vi "Read Cooler ON_OFF.vi"(8 "error in (no error)":errorcluster, 11 "CCDCamera in":refnum<class "Simulated_CCD_Camera.lvclass">) -> (0 "error out":errorcluster, 2 "COOLER_POWER_STATUS":u16, 3 "CCDCamera out":refnum<class "Simulated_CCD_Camera.lvclass">)   [LabVIEW 2018, in "Simulated_CCD_Camera.lvclass"]
uses:
  Simulated_CCD_Camera.lvclass
  Simulated_CCD_Camera.lvclass/Simulated_CCD_Camera.ctl
  Interface/Interface.lvclass
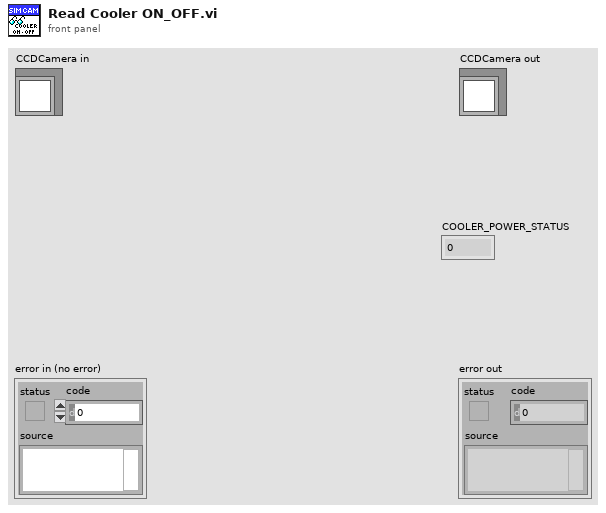
[diagram p1: front panel]
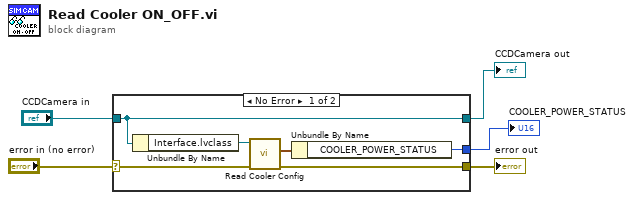
[diagram p0: block diagram]
diagram:
  n1 = case shown="No Error" "error in (no error)" {
    selector: "error in (no error)" -> [w10 w13]
    tunnel: [w7 w13] -> w4
    tunnel: [w11 w12] -> w2
    tunnel: "CCDCamera in" -> [w11 w12]
    tunnel: [w6 _] -> w1
    frame No Error {
      n2 = Unbundle By Name(w11) -> ("Interface.lvclass"=w9:refnum<class "Interface.lvclass">)
      n3 = call "Read Cooler Config.vi"("error in (no error)"=w10, "Interface in"=w9) -> ("error out"=w7:errorcluster, "Cooler Config"=w8:cluster{"COOLER_POWER_STATUS":u16, "TEMP":i32})  [unwired: 7 in, 1 out]
      n4 = Unbundle By Name(w8) -> ("COOLER_POWER_STATUS"=w6:u16)
    }
    frame Error {
    }
  }
  "error out" <- w4
  "CCDCamera out" <- w2
  "COOLER_POWER_STATUS" <- w1
